vi "Configure HSDIO Gen and Acq w_Waveform.vi"(7 "logic family":T1=8 items=["5.0V Logic"=5, "3.3V Logic"=6, "2.5V Logic"=7, "1.8V Logic"=8, "1.5V Logic"=80, "1.2V Logic"=81], 8 "error in (no error)":errorcluster, 9 "Clock Rate":dbl=20000000.0 format="%.2p", 10 "Pins":string[](array[string]), 11 "Semiconductor Module Context":T2) -> (0 "error out":errorcluster)   [LabVIEW 2013]
uses:
  <vilib>/NI_TestStand_SemiconductorModule/NI_TestStand_Semiconductor_Module.lvlibp/PinMap/General/SemiconductorModuleContext.ctl
  <instrlib>/niHSDIO/niHSDIO.llb/niHSDIO_ctl Voltage Logic Family Values (Ring).ctl
  <instrlib>/niHSDIO/niHSDIO.llb/niHSDIO_ctl Trigger Script - trigID Values (Ring).ctl
  <instrlib>/niHSDIO/niHSDIO.llb/niHSDIO_ctl Generation Mode Values (Ring).ctl
  <instrlib>/niHSDIO/niHSDIO.llb/niHSDIO_ctl Data Position Values (Ring).ctl
  <instrlib>/niHSDIO/niHSDIO.llb/niHSDIO_ctl Trigger Source Values (Ring).ctl
  <instrlib>/niHSDIO/niHSDIO.llb/niHSDIO_ctl Exported Signal Name Values (Ring).ctl
  <vilib>/NI_TestStand_SemiconductorModule/NI_TestStand_Semiconductor_Module.lvlibp/PinMap/HSDIO/PinsToNIHSDIOSessions.vi
  <instrlib>/niHSDIO/niHSDIO.llb/niHSDIO Configure Digital Edge Start Trigger.vi
  <instrlib>/niHSDIO/niHSDIO.llb/niHSDIO Configure Data Voltage Logic Family.vi
  <instrlib>/niHSDIO/niHSDIO.llb/niHSDIO Configure Software Script Trigger.vi
  <instrlib>/niHSDIO/niHSDIO.llb/niHSDIO Configure Initial State (String).vi
  <instrlib>/niHSDIO/niHSDIO.llb/niHSDIO Configure Idle State (String).vi
  <vilib>/NI_TestStand_SemiconductorModule/NI_TestStand_Semiconductor_Module.lvlibp
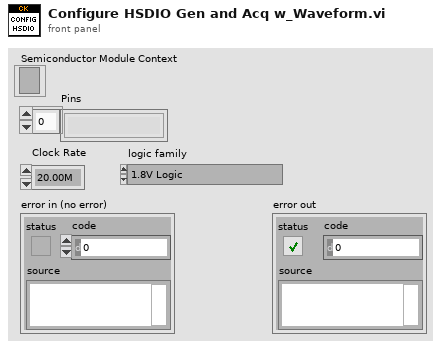
[diagram p1: front panel]
types:
  T1 = typedef "niHSDIO_ctl Voltage Logic Family Values (Ring).ctl" = i32
  T2 = typedef "NI_TestStand_Semiconductor_Module.lvlibp/SemiconductorModuleContext.ctl" = refnum<k7>
  T3 = typedef "niHSDIO_ctl Trigger Script - trigID Values (Ring).ctl" = string
  T4 = typedef "niHSDIO_ctl Exported Signal Name Values (Ring).ctl" = u16
  T5 = typedef "niHSDIO_ctl Trigger Source Values (Ring).ctl" = string
  T6 = typedef "niHSDIO_ctl Data Position Values (Ring).ctl" = i32
  T7 = typedef "niHSDIO_ctl Generation Mode Values (Ring).ctl" = i32
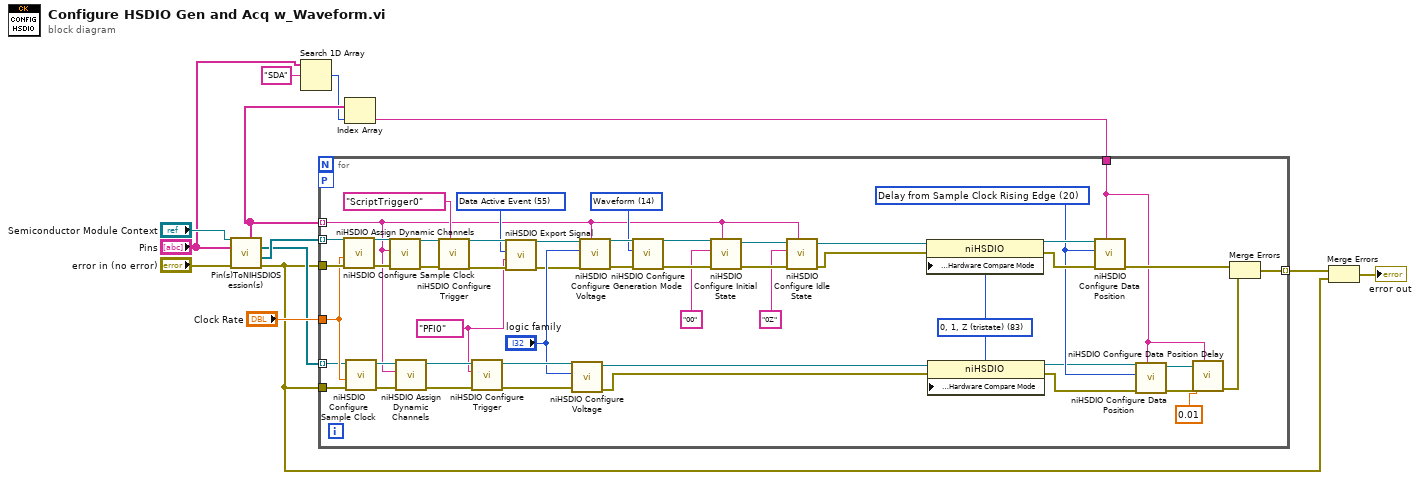
[diagram p0: block diagram]
diagram:
  n1 = call-poly <vilib>:"Pin(s)ToNIHSDIOSession(s).vi"("error in (no error)"="error in (no error)", "Pins"="Pins", "Semiconductor Module Context"="Semiconductor Module Context") -> ("error out"=w7:errorcluster, "Generation Sessions"=w13:refnum<k15>[], "Acquisition Sessions"=w8:refnum<k15>[], "Channel Lists"=w2:string[])  [unwired: 3 in, 2 out]
  n2 = Search 1D Array(1D array="Pins", element="SDA") -> (index of element=w1:i32)  [unwired: 1 in]
  n3 = Index Array(array=w2, index=w1) -> (element=w3:string)
  n4 = for {
    tunnel: w2 -> [w14] mode=indexing
    tunnel: w13 -> [w62] mode=indexing
    tunnel: "Clock Rate" -> [w51]
    workers-P: _ -> [_]
    tunnel: w7 -> [w63]
    tunnel: w8 -> [w50] mode=indexing
    tunnel: w7 -> [w49]
    tunnel: [w22] -> w6 mode=indexing
    tunnel: w3 -> [w21]
    w26 = T4 55 items=["Sample Clock"=51, "Reference Clock"=52, "Start Trigger"=53, "Reference Trigger"=54, "Advance Trigger"=61, "Pause Trigger"=57, "Script Trigger"=58, "Stop Trigger"=82, "Data Active Event"=55, "Marker Event"=59, "Ready For Start Event"=56, "Ready For Advance Event"=66, "End Of Record Event"=68, "Onboard Ref Clock"=60] ("signal (sample clock)")
    w25 = T5 "PFI0" ("source (PFI 0)")
    w39 = 83 items=["0, 1 (binary)"=77, "0, 1, Z (tristate)"=83, "0, 1, Z, L, H, X (stim/resp)"=78, "L, H, X (resp only)"=79] ("Advanced:Supported Data States")
    w35 = T6 20 items=["Sample Clock Rising Edge"=18, "Sample Clock Falling Edge"=19, "Delay from Sample Clock Rising Edge"=20] ("position (rising edge)")
    w54 = T7 14 items=["Waveform"=14, "Scripted"=15] ("generation mode (waveform)")
    n5 = call <instrlib>:"niHSDIO Configure Sample Clock.vi"("error in (no error)"=w63, "clock rate (50MHz)"=w51, "instrument handle"=w62) -> ("error out"=w61:errorcluster, "instrument handle out"=w60:refnum<k15>)  [unwired: 7 in]
    n6 = call <instrlib>:"niHSDIO Configure Sample Clock.vi"("error in (no error)"=w49, "clock rate (50MHz)"=w51, "instrument handle"=w50) -> ("error out"=w48:errorcluster, "instrument handle out"=w47:refnum<k15>)  [unwired: 7 in]
    n7 = call <instrlib>:"niHSDIO Assign Dynamic Channels.vi"("error in (no error)"=w61, "channel list (all:\"\")"=w14, "instrument handle"=w60) -> ("error out"=w59:errorcluster, "instrument handle out"=w58:refnum<k15>)  [unwired: 7 in]
    n8 = call <instrlib>:"niHSDIO Assign Dynamic Channels.vi"("error in (no error)"=w48, "channel list (all:\"\")"=w14, "instrument handle"=w47) -> ("error out"=w45:errorcluster, "instrument handle out"=w46:refnum<k15>)  [unwired: 7 in]
    n9 = call-poly <instrlib>:"niHSDIO Configure Trigger.vi"("trigger id (script trigger 0)"=T3 "ScriptTrigger0", "error in (no error)"=w59, "instrument handle"=w58) -> ("error out"=w27:errorcluster, "instrument handle out"=w30:refnum<k15>)  [unwired: 7 in]
    n10 = call-poly <instrlib>:"niHSDIO Configure Trigger.vi"("error in (no error)"=w45, "source (PFI 0)"=w25, "instrument handle"=w46) -> ("error out"=w44:errorcluster, "instrument handle out"=w43:refnum<k15>)  [unwired: 7 in]
    n11 = call <instrlib>:"niHSDIO Export Signal.vi"("error in (no error)"=w27, "output terminal (do not export)"=w25, "signal (sample clock)"=w26, "instrument handle"=w30) -> ("error out"=w28:errorcluster, "instrument handle out"=w29:refnum<k15>)  [unwired: 6 in]
    n12 = call-poly <instrlib>:"niHSDIO Configure Voltage.vi"("error in (no error)"=w44, "logic family (3.3V logic)"="logic family", "instrument handle"=w43) -> ("error out"=w37:errorcluster, "instrument handle out"=w38:refnum<k15>)  [unwired: 7 in]
    n13 = call-poly <instrlib>:"niHSDIO Configure Voltage.vi"("channel list (all:\"\")"=w14, "error in (no error)"=w28, "logic family (3.3V logic)"="logic family", "instrument handle"=w29) -> ("error out"=w56:errorcluster, "instrument handle out"=w55:refnum<k15>)  [unwired: 6 in]
    n14 = call <instrlib>:"niHSDIO Configure Generation Mode.vi"("error in (no error)"=w56, "generation mode (waveform)"=w54, "instrument handle"=w55) -> ("error out"=w53:errorcluster, "instrument handle out"=w52:refnum<k15>)  [unwired: 7 in]
    n15 = call-poly <instrlib>:"niHSDIO Configure Initial State.vi"("channel list"=w14, "error in (no error)"=w53, "initial state"="00", "instrument handle"=w52) -> ("error out"=w20:errorcluster, "instrument handle out"=w19:refnum<k15>)  [unwired: 6 in]
    n16 = call-poly <instrlib>:"niHSDIO Configure Idle State.vi"("channel list"=w14, "error in (no error)"=w20, "idle state"="0Z", "instrument handle"=w19) -> ("error out"=w16:errorcluster, "instrument handle out"=w15:refnum<k15>)  [unwired: 6 in]
    n17 = property on="Property Node" class="niHSDIO"(reference=w15, error in=w16, "Advanced:Hardware Compare:Hardware Compare Mode"=w39) -> (reference out=w41:refnum<k15>, error out=w40:errorcluster)
    n18 = property on="Property Node" class="niHSDIO"(reference=w38, error in=w37, "Advanced:Hardware Compare:Hardware Compare Mode"=w39) -> (reference out=w32:refnum<k15>, error out=w36:errorcluster)
    n19 = call <instrlib>:"niHSDIO Configure Data Position.vi"("channel list (all:\"\")"=w21, "error in (no error)"=w40, "position (rising edge)"=w35, "instrument handle"=w41) -> ("error out"=w24:errorcluster)  [unwired: 6 in, 1 out]
    n20 = call <instrlib>:"niHSDIO Configure Data Position.vi"("channel list (all:\"\")"=w21, "error in (no error)"=w36, "position (rising edge)"=w35, "instrument handle"=w32) -> ("error out"=w31:errorcluster, "instrument handle out"=w33:refnum<k15>)  [unwired: 6 in]
    n21 = call <instrlib>:"niHSDIO Configure Data Position Delay.vi"("channel list (all:\"\")"=w21, "error in (no error)"=w31, "delay (0.000)"=0.01, "instrument handle"=w33) -> ("error out"=w23:errorcluster)  [unwired: 6 in, 1 out]
    n22 = Merge Errors(w24, w23) -> (w22:errorcluster)
  }
  n23 = Merge Errors(w6, w7) -> (→"error out":errorcluster)
